vi "PyTest.vi"() -> ()   [LabVIEW 2020]
panel:
  out "Cutelog PID":i32
  in  "Stop Cutelog":bool caption="Blandadk Button"
  in  "Start Cutelog":bool caption="Blandadk Button"
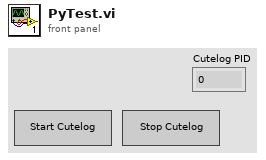
[diagram p1: front panel]
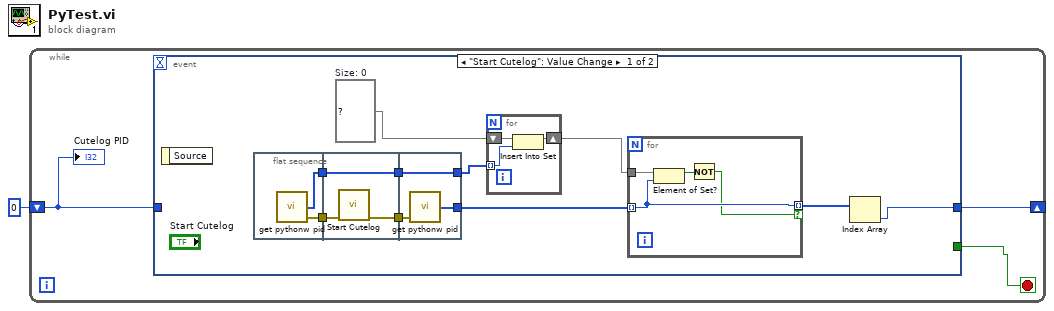
[diagram p0: block diagram]
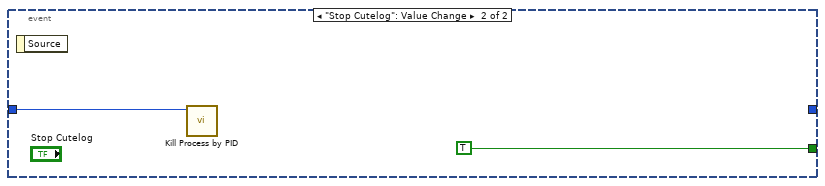
[diagram p2: hidden frame]
diagram:
  n1 = while {
    shift-right: [w4] -> _
    shift-left: 0 -> [w3]
    stop <- w2 stop-if-true
    n2 = event shown="[0] \"Start Cutelog\": Value Change" {
      selector: _ -> [_ _]
      dyn-events: _ -> [_ _]
      timeout: _ -> [_ _]
      tunnel: [w8 _] -> w4
      tunnel: w3 -> [_ w31]
      tunnel: [_ TRUE] -> w2
      event "Start Cutelog": Value Change {
        w7 = set{i32} {}  # Size: 0
        n3 = event-data() -> ()  [unwired: 1 in, 1 out]
        n4 = flat-sequence {
          tunnel: [w23] -> w14
          tunnel: [w22] -> w13
          tunnel: w14 -> [w25]
          tunnel: [w26] -> w12
          tunnel: [w24] -> w11
          tunnel: w13 -> [w24]
          tunnel: w12 -> [w29]
          tunnel: [w28] -> w6
          tunnel: w11 -> [w28]
          tunnel: [w27] -> w10
          frame #0 {
            n5 = call "get pythonw pid.vi"() -> ("error out"=w23:errorcluster, "PIDs"=w22:i32[])  [unwired: 4 in]
          }
          frame #1 {
            n6 = call "Start Cutelog.vi"("error in (no error)"=w25) -> ("error out"=w26:errorcluster)  [unwired: 10 in]
          }
          frame #2 {
            n7 = call "get pythonw pid.vi"("error in (no error)"=w29) -> ("PIDs"=w27:i32[])  [unwired: 3 in, 1 out]
          }
        }
        n8 = for {
          tunnel: w6 -> [w16] mode=indexing
          shift-right: [w15] -> w5
          shift-left: w7 -> [w17]
          n9 = Insert Into Set(10:w16, 11:w17) -> (3:w15:set{i32})  [unwired: 1 out]
        }
        n10 = for {
          tunnel: w10 -> [w19] mode=indexing
          tunnel: [w19] -> w9 mode=indexing if=w18
          tunnel: w5 -> [w21]
          n11 = Element of Set?(10:w19, 11:w21) -> (3:w20:bool)
          n12 = Not(x=w20) -> (.not. x?=w18:bool)
        }
        n13 = Index Array(array=w9) -> (element=w8:i32)  [unwired: 1 in]
      }
      event "Stop Cutelog": Value Change {
        n14 = event-data() -> ()  [unwired: 1 in, 1 out]
        n15 = call "Kill Process by PID.vi"("PID"=w31) -> ()  [unwired: 10 in, 1 out]
      }
    }
    "Cutelog PID" <- w3
  }
